vi "Read Measurement Values.vi"(6 "MeasurementListBox":refnum<vi>, 7 "Algo Override\nJSON Variant in":variant, 8 "error in":errorcluster, 9 "Read Edit Tolerance \nOverride JSON":path=path "C:/Users/raakeshs/Desktop/GTRON/Zengage 3.0/Configuration file/Gtron System JSON 2nd June 2017.json", 10 "Input ListBox Cluster":T1, 11 "Part Name in":string) -> (0 "error out":errorcluster, 2 "Number of\nMeasurements":u8, 3 "ListBox Cluster out":T1)   [LabVIEW 2019, in "ZenGage v3.0 UI.lvclass"]
uses:
  ZenGage v3.0 UI.lvclass
  <vilib>/Utility/miscctls.llb/LVRowAndColumnTypeDef.ctl
  Type Definitions/Edit tolerance settings/Edit Tolerance Input.ctl
  Type Definitions/Edit tolerance settings/Rack Selection.ctl
  <vilib>/Utility/miscctls.llb/LVPoint32TypeDef.ctl
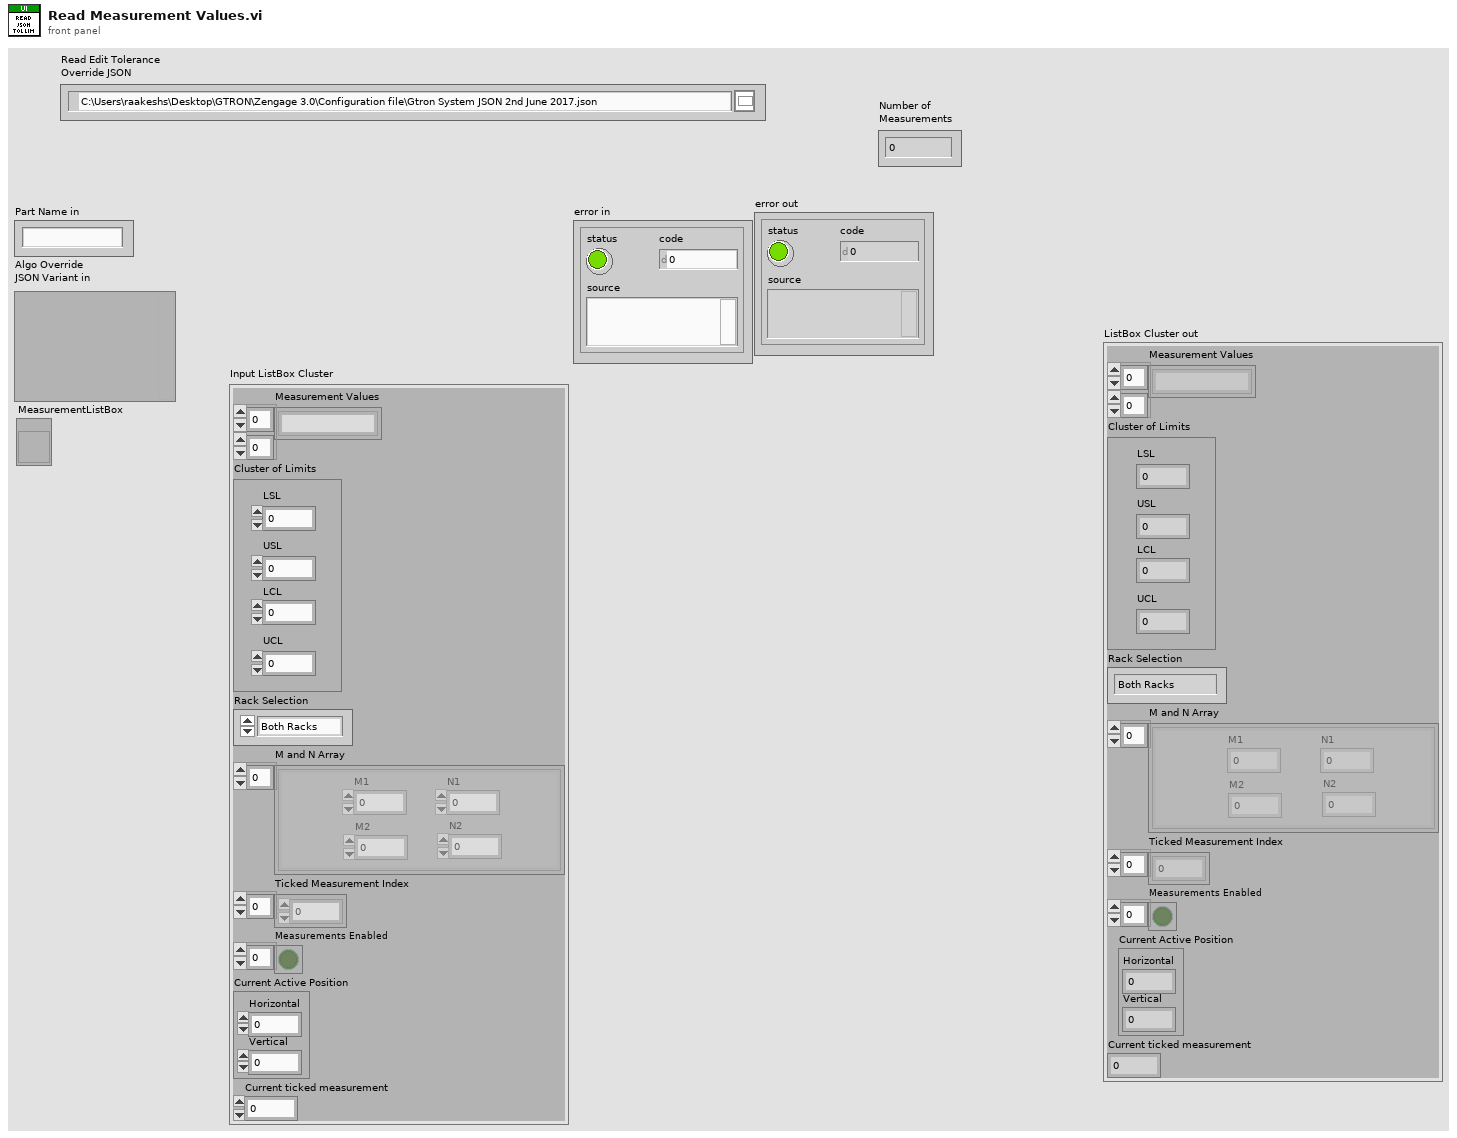
[diagram p1: front panel]
types:
  T1 = typedef "ZenGage v3.0 UI.lvclass/Edit Tolerance Input.ctl" = cluster{"Measurement Values":string[][], "Cluster of Limits":cluster{"LSL":dbl, "USL":dbl, "LCL":dbl, "UCL":dbl}, "Rack Selection":T2, "M and N Array":cluster{"M1":u64, "M2":u64, "N1":u64, "N2":u64}[], "Ticked Measurement Index":u32[], "Measurements Enabled":bool[], "Current Active Position":T3, "Current ticked measurement":dbl}
  T2 = typedef "ZenGage v3.0 UI.lvclass/Rack Selection.ctl" = enum16{"Both Racks", "Rack 2", "Rack 1"}
  T3 = typedef "LVPoint32TypeDef.ctl" = cluster{"Horizontal":i32, "Vertical":i32}
  T4 = enum8{"Enabled", "Disabled", "Disabled and Grayed Out"}
  T5 = cluster{"Name":string, "Measurements":cluster{"RackID":i32, "MeasurementId":i32, "Name":string, "AlgoName":string, "MeasurementEnable":bool, "Calibration Coefficients":cluster{"Linearity Correction":dbl, "Bias Correction":dbl}, "SpecValues":cluster{"LCL":dbl, "UCL":dbl, "LSL":dbl, "USL":dbl, "NominalValue":dbl}}[]}
  T6 = cluster{"RackID":i32, "MeasurementId":i32, "Name":string, "AlgoName":string, "MeasurementEnable":bool, "Calibration Coefficients":cluster{"Linearity Correction":dbl, "Bias Correction":dbl}, "SpecValues":cluster{"LCL":dbl, "UCL":dbl, "LSL":dbl, "USL":dbl, "NominalValue":dbl}}[]
  T7 = typedef "LVRowAndColumnTypeDef.ctl" = cluster{"Row":i32, "Column":i32}
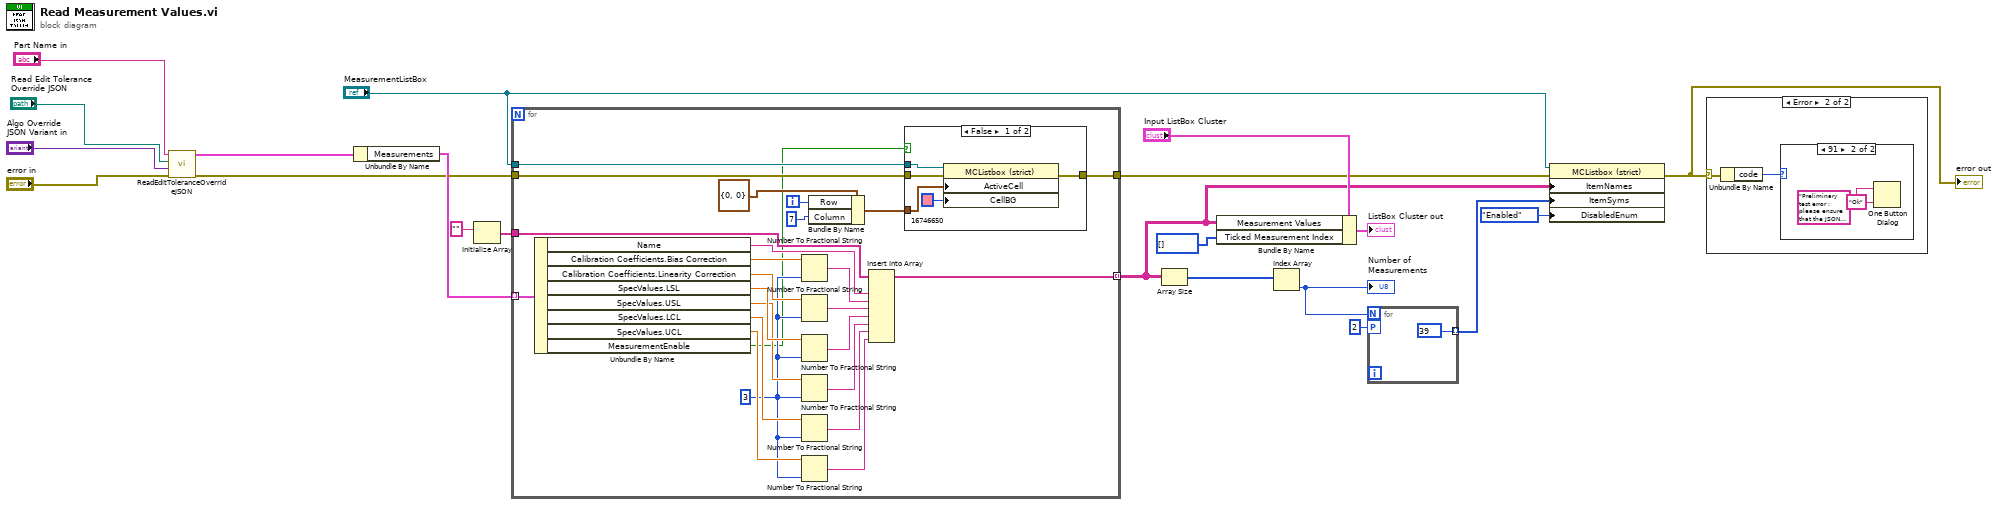
[diagram p0: block diagram]
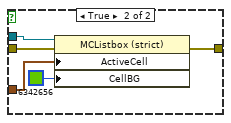
[diagram p4: hidden frame]
diagram:
  n1 = call "ReadEditToleranceOverrideJSON.vi"("error in"="error in", "Algo Override\nJSON Variant in"="Algo Override\nJSON Variant in", "Read Edit Tolerance \nOverride JSON"="Read Edit Tolerance \nOverride JSON", "Part Name"="Part Name in") -> ("error out"=w5:errorcluster, "Cluster"=w21:T5)  [unwired: 6 in]
  n2 = Unbundle By Name(w21) -> ("Measurements"=w20:T6)
  n3 = Initialize Array("") -> (w18:string[])  [unwired: 1 in]
  n4 = for {
    tunnel: w20 -> [w46] mode=indexing
    tunnel: w18 -> [w43]
    tunnel: [w44] -> w9 mode=indexing
    tunnel: w5 -> [w24]
    tunnel: [w23] -> w4
    tunnel: "MeasurementListBox" -> [w39]
    i -> [w25]
    w32 = i16 3 ("width (-)")
    n5 = Unbundle By Name(w46) -> ("Name"=w45:string, "Calibration Coefficients.Bias Correction"=w38:dbl, "Calibration Coefficients.Linearity Correction"=w37:dbl, "SpecValues.LSL"=w36:dbl, "SpecValues.USL"=w35:dbl, "SpecValues.LCL"=w34:dbl, "SpecValues.UCL"=w33:dbl, "MeasurementEnable"=w22:bool)
    n6 = Number To Fractional String(number=w38, precision (6)=w32) -> (F-format string=w31:string)  [unwired: 2 in]
    n7 = Number To Fractional String(number=w37, precision (6)=w32) -> (F-format string=w30:string)  [unwired: 2 in]
    n8 = Number To Fractional String(number=w36, precision (6)=w32) -> (F-format string=w29:string)  [unwired: 2 in]
    n9 = Number To Fractional String(number=w35, precision (6)=w32) -> (F-format string=w28:string)  [unwired: 2 in]
    n10 = Number To Fractional String(number=w34, precision (6)=w32) -> (F-format string=w27:string)  [unwired: 2 in]
    n11 = Number To Fractional String(number=w33, precision (6)=w32) -> (F-format string=w26:string)  [unwired: 2 in]
    n12 = Bundle By Name(cluster=T7 {"Row"=0, "Column"=0} ("Active Cell:Active Cell"), "Row"=w25, "Column"=7) -> (w40:T7)
    n13 = Insert Into Array(array=w43, new element #1=w45, new element #2=w31, new element #3=w30, new element #4=w29, new element #5=w28, new element #6=w27, new element #7=w26) -> (w44:string[])  [unwired: 1 in]
    n14 = case shown="False" w22 {
      tunnel: w40 -> [w51 w56]
      tunnel: w24 -> [w50 w55]
      tunnel: [w49 w54] -> w23
      tunnel: w39 -> [w48 w53]
      frame False {
        n15 = property class="MCListbox (strict)"(reference=w48, error in=w50, "ActiveCell"=w51, "CellBG"=u32 16746650) -> (error out=w49:errorcluster)  [unwired: 1 out]
      }
      frame True {
        n16 = property class="MCListbox (strict)"(reference=w53, error in=w55, "ActiveCell"=w56, "CellBG"=u32 6342656) -> (error out=w54:errorcluster)  [unwired: 1 out]
      }
    }
  }
  n17 = Array Size(array=w9) -> (size(s)=w12:i32[])
  n18 = Bundle By Name(cluster="Input ListBox Cluster", "Measurement Values"=w9, "Ticked Measurement Index"=u32[] [] ("Input Data Cluster.Ticked Measurement Index")) -> (→"ListBox Cluster out":T1)
  n19 = Index Array(array=w12) -> (element=w11:i32)  [unwired: 1 in]
  "Number of\nMeasurements" <- w11
  n20 = for {
    N: w11 -> [_]
    tunnel: [39] -> w10 mode=indexing
    workers-P: 2 -> [_]
  }
  n21 = property class="MCListbox (strict)"(reference="MeasurementListBox", error in=w4, "ItemNames"=w9, "ItemSyms"=w10, "DisabledEnum"=T4."Enabled" ("Disabled")) -> (error out=w1:errorcluster)  [unwired: 1 out]
  "error out" <- w1
  n22 = case shown="Error" w1 {
    selector: w1 -> [_ w59]
    frame No Error {
    }
    frame Error {
      n23 = Unbundle By Name(w59) -> ("code"=w58:i32)
      n24 = case shown="91" w58 {
        frame 0, Default {
        }
        frame 91 {
          n25 = One Button Dialog(message="Preliminary test error : please ensure that the JSON configuration structure has not been modified. If yes, then please modify the algorithm override typedef in the user interface module.\nIt is recommended to exit the software now. ", button name ("OK")="Ok") -> ()  [unwired: 1 out]
        }
      }
    }
  }
